vi "zlgcan_demo_CANET_UDP.vi"() -> ()   [LabVIEW 2018]
doc: "适用的设备：CANET-E-U、CANET-2E-U、CANET-4E-U、CANET-8E-U、\nCANET-200T、CANET-100T"
uses:
  data_type/ZCAN_Transmit_Data.ctl
panel:
  in  "本地端口":u32=8000
  in  "工作端口":u32=4001
  in  "IP":string="192.168.0.178"
  in  "CANFD数据帧数组":T1(array[cluster])
  in  "CAN数据帧数组":T2(array[cluster])
  out "已接收帧数":u32
  out "CAN报文显示":string[][](table)
  out "CANFD报文显示":string[][](table)
  out "error out 2":errorcluster caption="错误输出"
  out "source":string
  in  "开启CAN":bool
  in  "stop":bool
  in  "?":T3(tab)
  in  "CAN卡型号":u32(ring)=12 items=["CANET-UDP"=12]
  in  "索引":u32(ring) items=["0", "1", "2", "3", "4", "5", "6", "7", "8"]
  in  "CAN 通道":u32(ring) items=["0", "1", "2", "3"]
  out "设备句柄":u32
  out "通道句柄":u32
  out "error out":errorcluster caption="状态"
  in  "帧类型":u32(ring) items=["标准帧", "扩展帧"]
  in  "发送方式":u32(ring) items=["正常发送", "单次发送", "自发自收", "单次自发自收"]
  in  "帧格式":u32(ring) items=["数据帧", "远程帧"]
  out "数据长度":u8=8 max=8
  in  "ID":u32=18 format="0x%08x"
  in  "协议":u32(ring) items=["CAN"]
  in  "数据输入":string="11 22 33 44 55 66 77 88"
  in  "发送":bool
  in  "ZCAN_Transmit_Data":T4
  # "适用的设备：CANET-E-U、CANET-2E-U、CANET-4E-U、\nCANET-8E-U、CANET-200T、CANET-100T"
  # "停止程序前，\n请先关闭CAN卡"
  # "当CANET的工作模式为：\n\n1. 客户端（TCP Client）\n\n   LabVIEW 设备型号选择【 CANET-TCP】\n\n   TCP模式选择【服务器 TCP Sever】\n\n   填写电脑本机IP+本地端口。\n\n2. 服务器（TCP Sever）\n\n   LabVIEW 设备型号选择【 CANET-TCP】\n\n   TCP模式选择【客户端 TCP Client】\n\n   填写CANET的 IP +工作端口\n\n3. UDP\n\n   LabVIEW 设备型号选择【 CANET-UDP】\n\n   填写CANET的IP+工作端口+本地端口"
  # "1. 调试运行DEMO前，将bin文件夹下面的kerneldlls文件夹先拷贝至LabView安装目录，\n如 D:\\Program Files (x86)\\National Instruments\\LabVIEW 2018。"
  # "2. 确保电脑有VC++ 2005/2008/2010/2013运行库（对应32，64位），可到微软官网下载。"
  # "3，如果打开设备失败，可能原因：\n（1）没有进行第二步操作；\n（2）已经打开过一次，没有正常关闭的情况下，继续点击“打开设备”，是无法打开的。\n     需要USB重新拔插，LABVIEW重启（全部关闭），然后再“打开设备”。\n (3) 项目路径不能有中文繁体。"
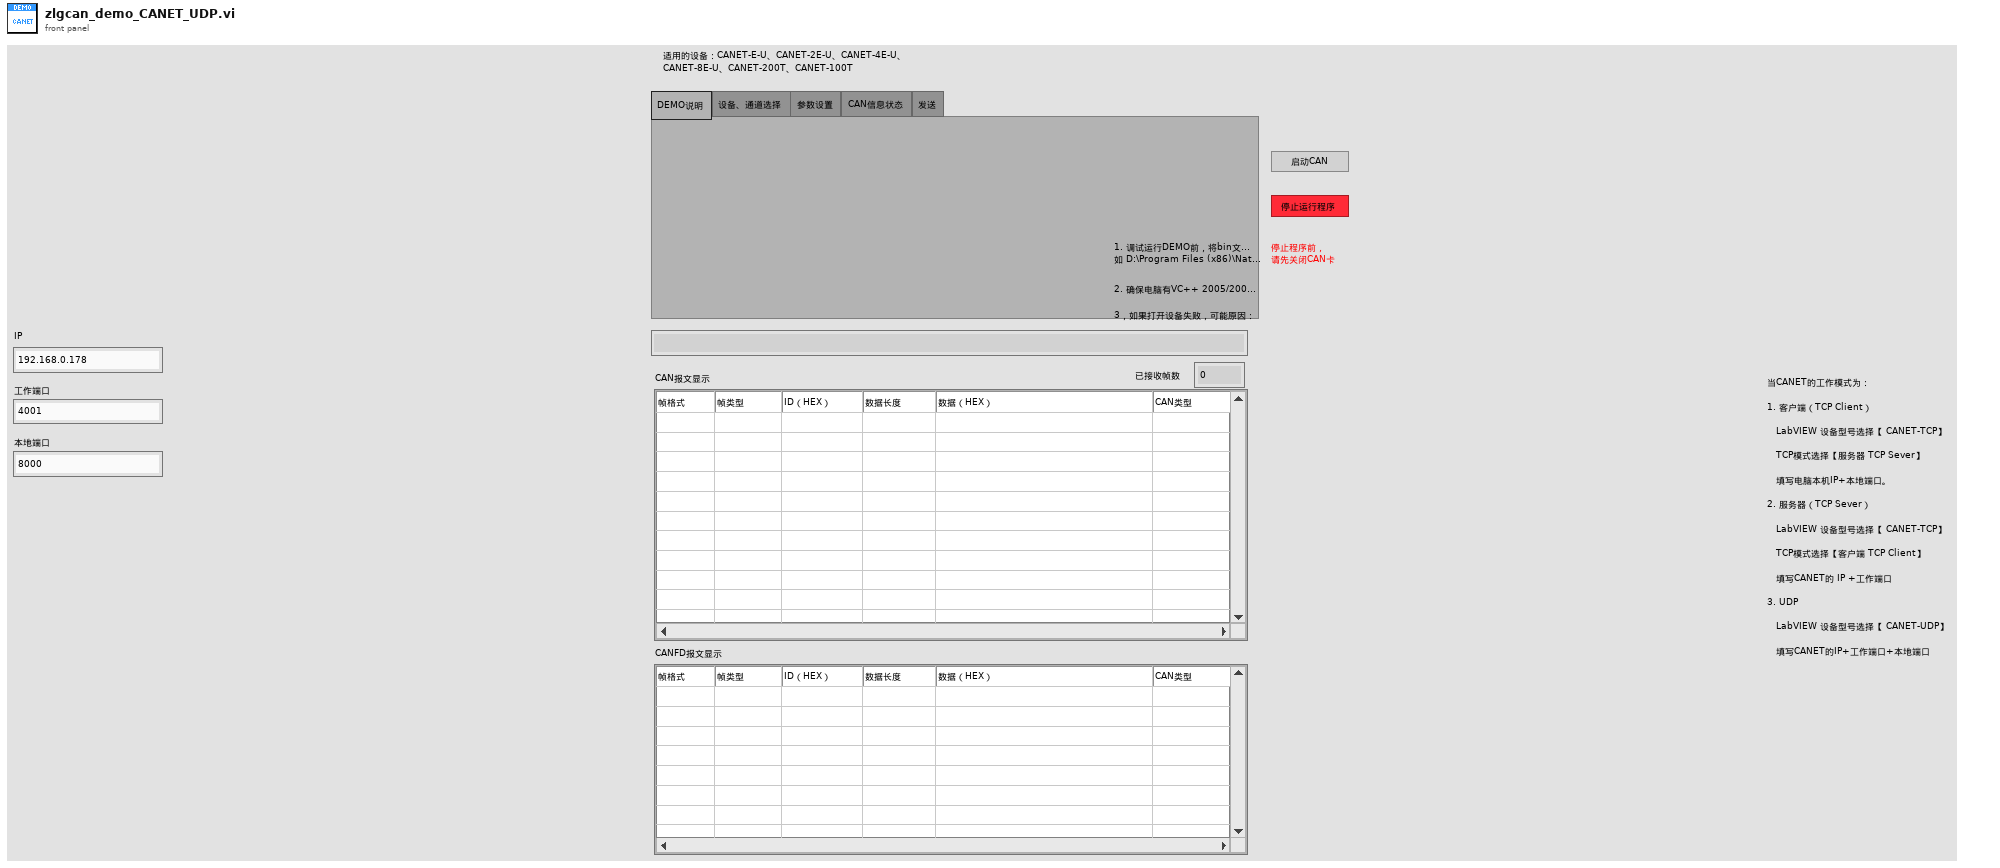
[diagram p1: front panel]
types:
  T1 = cluster{u32, u8, u8, u8, u8, cluster{"[0]":u8, "[1]":u8, "[2]":u8, "[3]":u8, "[4]":u8, "[5]":u8, "[6]":u8, "[7]":u8, "[8]":u8, "[9]":u8, "[10]":u8, "[11]":u8, "[12]":u8, "[13]":u8, "[14]":u8, "[15]":u8, "[16]":u8, "[17]":u8, "[18]":u8, "[19]":u8, "[20]":u8, "[21]":u8, "[22]":u8, "[23]":u8, "[24]":u8, "[25]":u8, "[26]":u8, "[27]":u8, "[28]":u8, "[29]":u8, "[30]":u8, "[31]":u8, "[32]":u8, "[33]":u8, "[34]":u8, "[35]":u8, "[36]":u8, "[37]":u8, "[38]":u8, "[39]":u8, "[40]":u8, "[41]":u8, "[42]":u8, "[43]":u8, "[44]":u8, "[45]":u8, "[46]":u8, "[47]":u8, "[48]":u8, "[49]":u8, "[50]":u8, "[51]":u8, "[52]":u8, "[53]":u8, "[54]":u8, "[55]":u8, "[56]":u8, "[57]":u8, "[58]":u8, "[59]":u8, "[60]":u8, "[61]":u8, "[62]":u8, "[63]":u8}, u64}[]
  T2 = cluster{u32, u8, u8, u8, u8, cluster{"[0]":u8, "[1]":u8, "[2]":u8, "[3]":u8, "[4]":u8, "[5]":u8, "[6]":u8, "[7]":u8}, u64}[]
  T3 = enum32{"DEMO说明", "设备、通道选择", "参数设置", "CAN信息状态", "发送"}
  T4 = typedef "ZCAN_Transmit_Data.ctl" = cluster{"帧类型":u32, "帧格式":u32, "ID":u32, "数据长度":u8, "DATA":cluster{"CAN数据[0]":u8, "CAN数据[1]":u8, "CAN数据[2]":u8, "CAN数据[3]":u8, "CAN数据[4]":u8, "CAN数据[5]":u8, "CAN数据[6]":u8, "CAN数据[7]":u8}, "发送方式":u32}
  T5 = cluster{"can_type":u32, "can_type":u32, "can_type":u32, "can_type":u32, "can_type":u8, "can_type":u8, "can_type":u8, "can_type":u8}
  T6 = cluster{"[0]":u32, "[1]":u32, "[2]":u32, "[3]":u32, "[4]":u32, "[5]":u32, "[6]":u32, "[7]":u32}
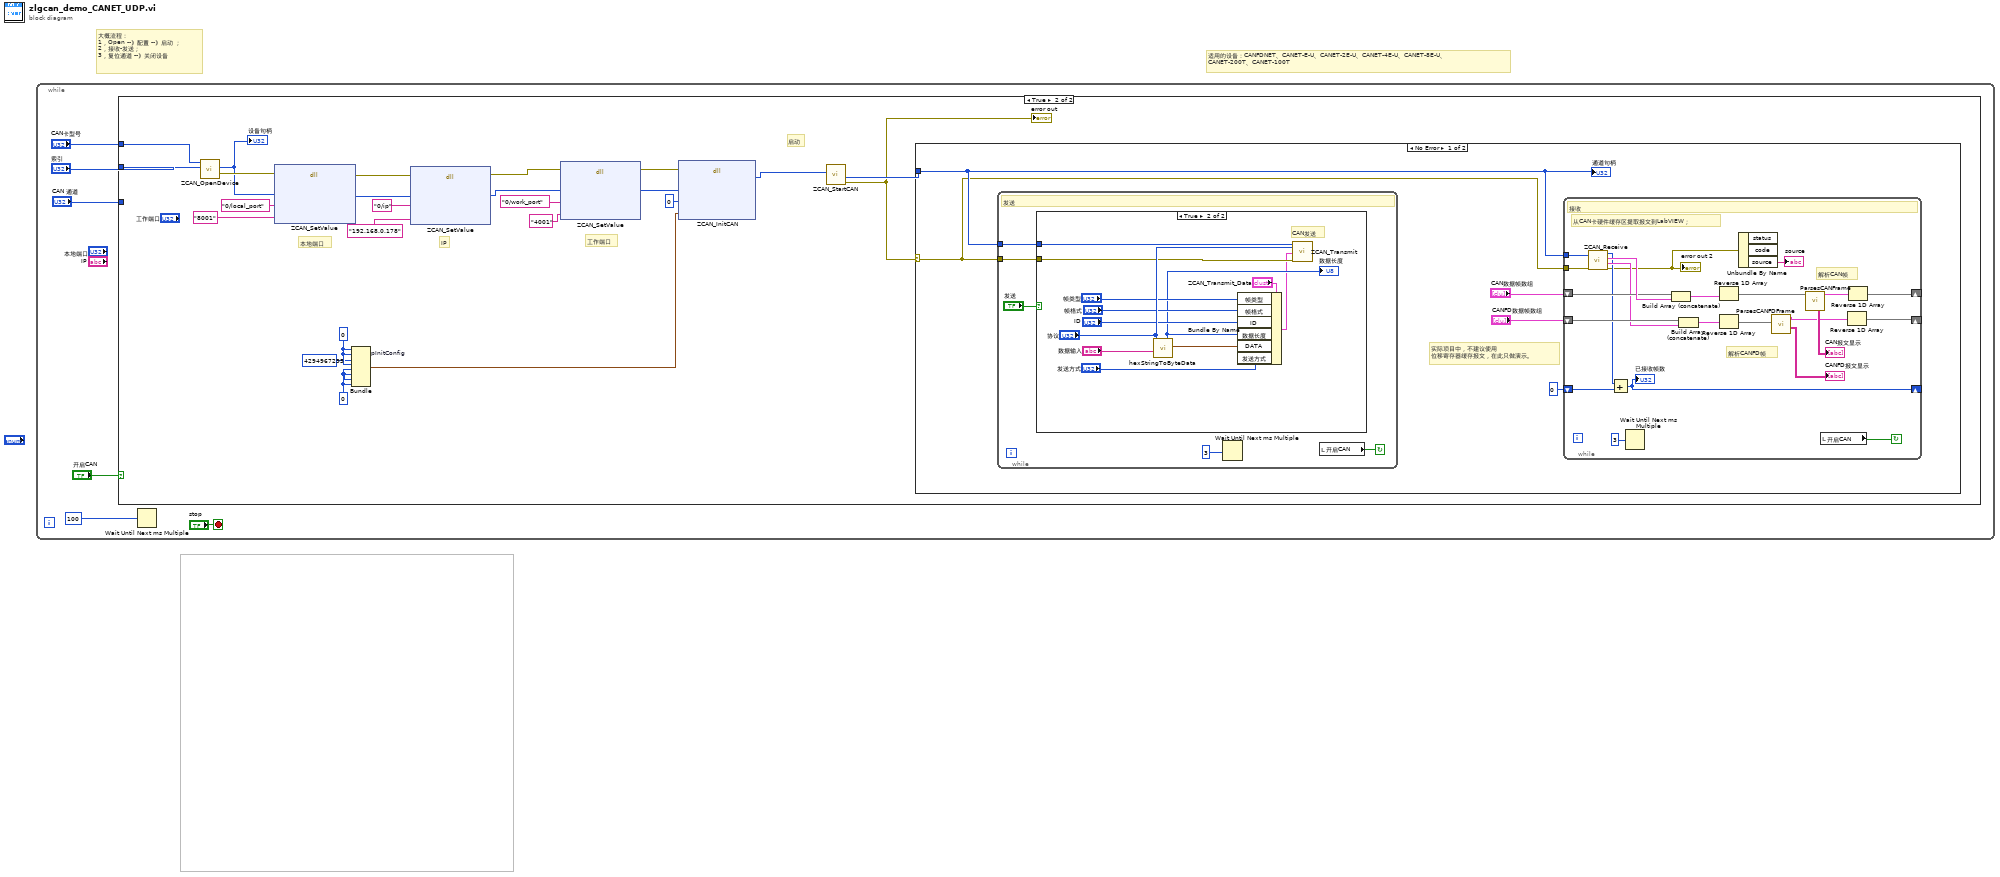
[diagram p0: block diagram]
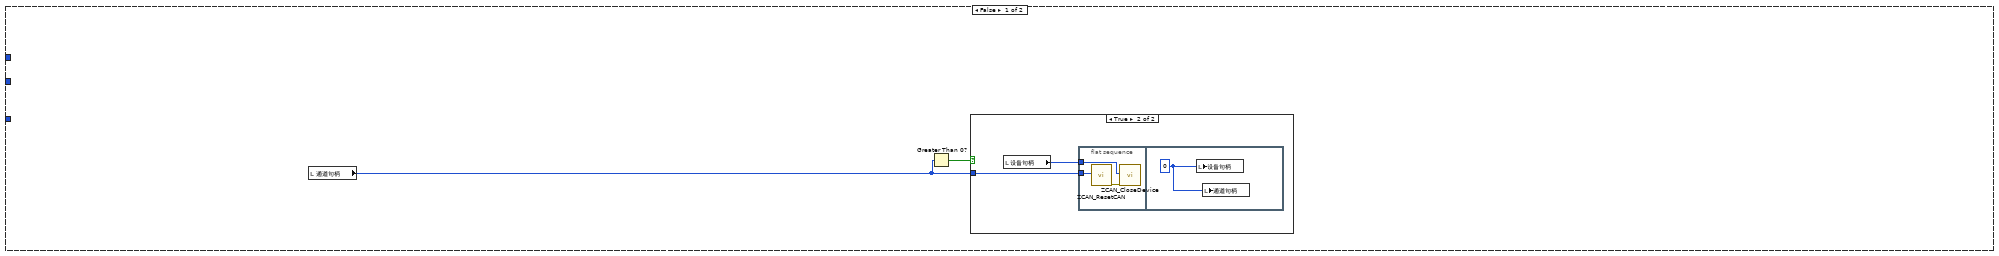
[diagram p2: hidden frame]
diagram:
  # "适用的设备：CANFDNET、CANET-E-U、CANET-2E-U、CANET-4E-U、CANET-8E-U、\nCANET-200T、CANET-100T"
  # "大概流程：\n1，Open --》配置 --》启动 ；\n2，接收-发送；\n3，复位通道 --》关闭设备"
  n1 = while {
    stop <- "stop" stop-if-true
    n2 = case shown="True" "开启CAN" {
      tunnel: "CAN卡型号" -> [_ w35]
      tunnel: "索引" -> [_ w38]
      tunnel: "CAN 通道" -> [_ _]
      frame False {
        # "关闭CAN卡"
        n3 = local read "通道句柄"() -> (w7:u32)
        n4 = Greater Than 0?(x=w7) -> (x > 0?=w8:bool)
        n5 = case shown="True" w8 {
          tunnel: w7 -> [_ w10]
          frame False {
          }
          frame True {
            n6 = local read "设备句柄"() -> (w9:u32)
            n7 = flat-sequence {
              tunnel: w10 -> [w12]
              tunnel: w9 -> [w11]
              frame #0 {
                n8 = call "ZCAN_ResetCAN.vi"("can_handle"=w12) -> ("error out"=w13:errorcluster)  [unwired: 9 in, 1 out]
                n9 = call "ZCAN_CloseDevice.vi"("error in (no error)"=w13, "device_handle"=w11) -> ()  [unwired: 8 in, 2 out]
              }
              frame #1 {
                w14 = u32 0 ("can_index_handle(out)")
                n10 = local write "设备句柄"(w14) -> ()
                n11 = local write "通道句柄"(w14) -> ()
              }
            }
          }
        }
      }
      frame True {
        w16 = u8 0 ("can_type")
        w18 = u32 0 ("can_type")
        # "工作端口"
        # "IP"
        # "启动"
        # "本地端口"
        n12 = call "ZCAN_OpenDevice.vi"("device_index"=w38, "device_type"=w35) -> ("error out"=w24:errorcluster, "DEVICE_HANDLE"=w23:u32)  [unwired: 8 in]
        "设备句柄" <- w23
        n13 = dll-call lib="PTH2oabs CUsersadminDesktop'完善2020版本zlgcan_labview_20220510zlgcan_demo_CANET_UDPbin\nzlgcan.dll" fn="ZCAN_SetValue"(error in=w24, "hDev"=w23, "path"="0/local_port", "value"="8001") -> (error out=w26:errorcluster, "hDev"=w31:u32)  [unwired: 5 in, 1 out]
        n14 = Bundle "pInitConfig"("can_type"=w18, "can_type"=w18, "can_type"=u32 4294967295, "can_type"=w18, "can_type"=w16, "can_type"=w16, "can_type"=w16, "can_type"=w16) -> (w19:T5)  [unwired: 1 in]
        n15 = dll-call lib="PTH2oabs CUsersadminDesktop'完善2020版本zlgcan_labview_20220510zlgcan_demo_CANET_UDPbin\nzlgcan.dll" fn="ZCAN_SetValue"(error in=w26, "hDev"=w31, "path"="0/ip", "value"="192.168.0.178") -> (error out=w25:errorcluster, "hDev"=w27:u32)  [unwired: 5 in, 1 out]
        n16 = dll-call lib="PTH2oabs CUsersadminDesktop'完善2020版本zlgcan_labview_20220510zlgcan_demo_CANET_UDPbin\nzlgcan.dll" fn="ZCAN_SetValue"(error in=w25, "hDev"=w27, "path"="0/work_port", "value"="4001") -> (error out=w22:errorcluster, "hDev"=w21:u32)  [unwired: 5 in, 1 out]
        n17 = dll-call lib="PTH2tabs CUsersadminDesktop'完善2020版本zlgcan_labview_20220510zlgcan_demo_CANET_UDPbinzlgcan_wrap.dll" fn="ZCAN_InitCAN"(error in=w22, "device_handle"=w21, "can_index"=0, "pInitConfig"=w19) -> ("can_handle"=w15:u32)  [unwired: 5 in, 2 out]
        n18 = call "ZCAN_StartCAN.vi"("can_index_handle"=w15) -> ("error out"=w36:errorcluster, "can_index_handle(out)"=w37:u32)  [unwired: 8 in, 1 out]
        "error out" <- w36
        n19 = case shown="No Error" w36 {
          selector: w36 -> [w39 _]
          tunnel: w37 -> [w40 _]
          frame No Error {
            # "实际项目中，不建议使用\n位移寄存器缓存报文，在此只做演示。"
            n20 = while {
              tunnel: w40 -> [w69]
              tunnel: w39 -> [w67]
              stop <- w68 continue-if-true
              # "发送"
              n21 = case shown="True" "发送" {
                tunnel: w69 -> [_ w76]
                tunnel: w67 -> [_ w77]
                frame False {
                }
                frame True {
                  # "CAN发送"
                  n22 = call "hexStringToByteData.vi"("数据输入"="数据输入", "协议"="协议") -> ("CAN_data"=w73:T6, "字节数"=w78:i32)  [unwired: 7 in, 1 out]
                  "数据长度" <- w78
                  n23 = Bundle By Name(cluster="ZCAN_Transmit_Data", "帧类型"="帧类型", "帧格式"="帧格式", "ID"="ID", "数据长度"=w78, "DATA"=w73, "发送方式"="发送方式") -> (w72:T4)
                  n24 = call "ZCAN_Transmit.vi"("can_index_handle"=w76, "协议"="协议", "ZCAN_Transmit_Data"=w72, "error in (no error)"=w77) -> ()  [unwired: 15 in, 1 out]
                }
              }
              n25 = Wait Until Next ms Multiple(millisecond multiple=u32 3) -> ()  [unwired: 1 out]
              n26 = local read "开启CAN"() -> (w68:bool)
            }
            n27 = while {
              tunnel: w39 -> [w64]
              tunnel: w40 -> [w63]
              shift-right: [w65] -> _
              shift-left: 0 -> [w51]
              shift-right: [w55] -> _
              shift-left: "CAN数据帧数组" -> [w61]
              shift-right: [w53] -> _
              shift-left: "CANFD数据帧数组" -> [w59]
              stop <- w44 continue-if-true
              # "从CAN卡硬件缓存区提取报文到LabVIEW；"
              # "解析CANFD帧"
              # "解析CAN帧"
              # "接收"
              n28 = call "ZCAN_Receive.vi"("error in (no error)"=w64, "can_handle"=w63) -> ("error out"=w45:errorcluster, "CANFD数据帧数组"=w58:T1, "CAN数据帧数组"=w62:T2, "Receive_Num"=w52:u32)  [unwired: 2 in]
              "error out 2" <- w45
              n29 = Add(x=w52, y=w51) -> (x+y=w65:u32)
              "已接收帧数" <- w65
              n30 = Wait Until Next ms Multiple(millisecond multiple=u32 3) -> ()  [unwired: 1 out]
              n31 = Build Array (concatenate)(w61, w62) -> (w60:T2)
              n32 = Build Array (concatenate)(w59, w58) -> (w57:T1)
              n33 = Reverse 1D Array(array=w60) -> (reversed array=w54:T2)
              n34 = Reverse 1D Array(array=w57) -> (reversed array=w49:T1)
              n35 = Unbundle By Name(w45) -> ("source"=→"source":string)  [unwired: 2 out]
              n36 = call "ParsesCANFDFrame.vi"("CANFD数据帧数组"=w49) -> ("CANFD报文显示"=→"CANFD报文显示":string[][], "CANFD数据帧数组(out)"=w48:T1)  [unwired: 9 in]
              n37 = call "ParsesCANFrame.vi"("CAN数据帧数组"=w54) -> ("CAN数据帧数组(out)"=w56:T2, "CAN报文显示"=→"CAN报文显示":string[][])  [unwired: 9 in]
              n38 = local read "开启CAN"() -> (w44:bool)
              n39 = Reverse 1D Array(array=w48) -> (reversed array=w53:T1)
              n40 = Reverse 1D Array(array=w56) -> (reversed array=w55:T2)
            }
            "通道句柄" <- w40
          }
          frame Error {
          }
        }
      }
    }
    n41 = Wait Until Next ms Multiple(millisecond multiple=u32 100) -> ()  [unwired: 1 out]
  }
